vi "CtrlTrain_Analog_Scale.vi"(4 "Raw_High":dbl=5.0, 6 "Raw_Low":dbl, 8 "Out_Low":dbl, 9 "Out_High":dbl=100.0, 11 "Input":dbl) -> (0 "B":dbl, 1 "M":dbl, 3 "Output":dbl)   [LabVIEW 2019, in "CtrlTrainingLibary_Protected.lvlib"]
doc: "This VI rate limits the input. This VI remembers the last output. If there are multiple VI that set the same output, use the RateLimit2 VI. This one has an input connection to send the last output value."
uses:
  CtrlTrainingLibary_Protected.lvlib
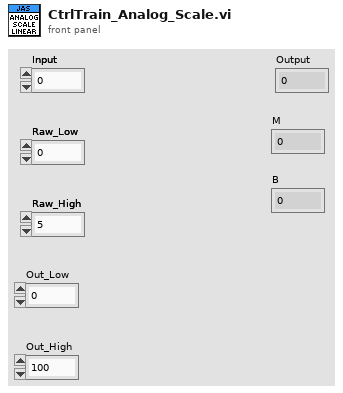
[diagram p1: front panel]
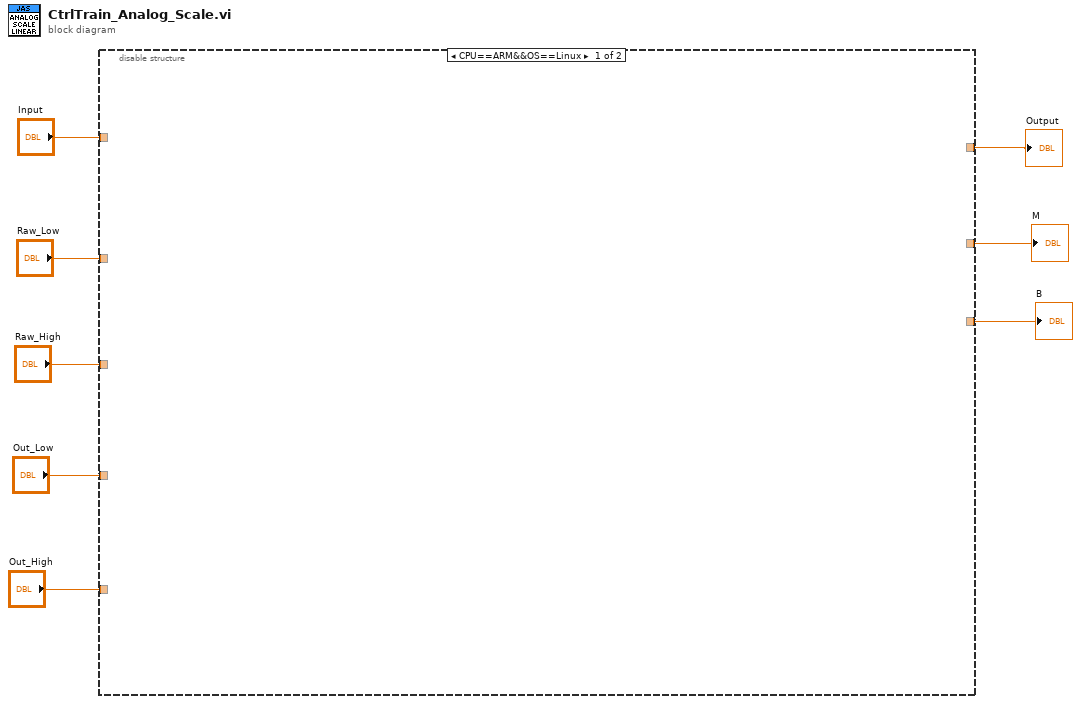
[diagram p0: block diagram]
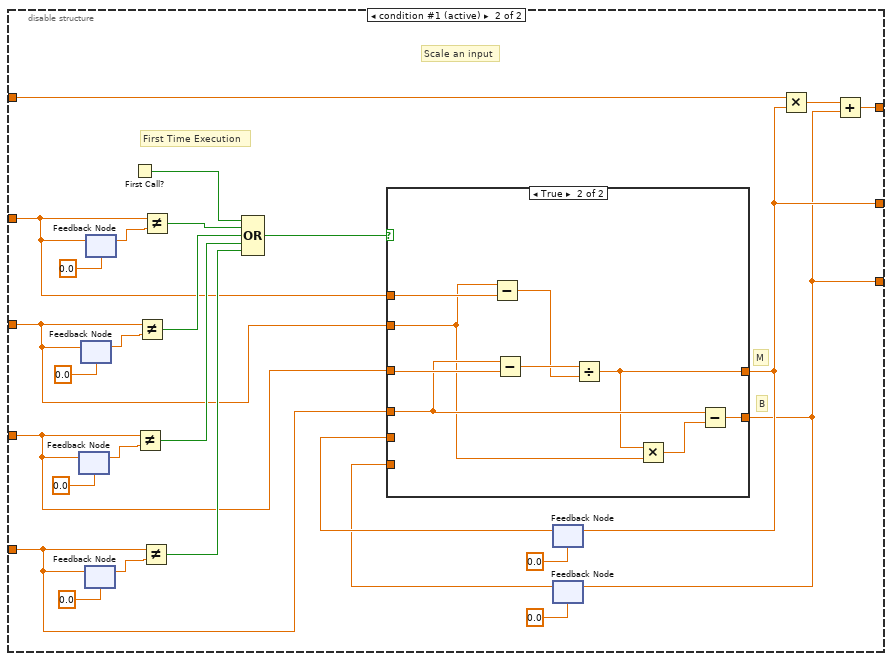
[diagram p2: hidden frame]
diagram:
  n1 = disable-structure shown="CPU==ARM&&OS==Linux" {
    disable-tunnel: "Raw_Low" -> [_ w22]
    disable-tunnel: "Raw_High" -> [_ w21]
    disable-tunnel: "Out_Low" -> [_ w20]
    disable-tunnel: "Out_High" -> [_ w19]
    disable-tunnel: "Input" -> [_ w18]
    disable-tunnel: [_ w16] -> w3
    disable-tunnel: [_ w13] -> w2
    disable-tunnel: [_ w10] -> w1
    frame condition #0 {
    }
    frame condition #1 (active) {
      # "First Time Execution"
      # "Scale an input"
      # "B"
      # "M"
      n2 = feedback #1(0.0 ("Raw_Low")) -> (w31:dbl)
      n3 = feedback-in #1(w20) -> ()
      n4 = feedback #2(0.0 ("Raw_Low")) -> (w33:dbl)
      n5 = feedback-in #2(w21) -> ()
      n6 = feedback #3(0.0 ("Raw_Low")) -> (w29:dbl)
      n7 = feedback-in #3(w19) -> ()
      n8 = feedback #4(0.0 ("Raw_Low")) -> (w35:dbl)
      n9 = feedback-in #4(w22) -> ()
      n10 = First Call?() -> (First Call?: T/F=w9:bool)
      n11 = Not Equal?(x=w20, y=w31) -> (x != y?=w25:bool)
      n12 = Not Equal?(x=w21, y=w33) -> (x != y?=w26:bool)
      n13 = Not Equal?(x=w19, y=w29) -> (x != y?=w24:bool)
      n14 = Not Equal?(x=w22, y=w35) -> (x != y?=w27:bool)
      n15 = Compound Arithmetic op=OR(w9, w27, w26, w25, w24) -> (w23:bool)
      n16 = feedback #5(0.0) -> (w12:dbl)
      n17 = feedback #6(0.0) -> (w11:dbl)
      n18 = case shown="True" w23 {
        tunnel: w22 -> [_ w45]
        tunnel: w21 -> [_ w41]
        tunnel: w20 -> [_ w46]
        tunnel: w19 -> [_ w42]
        tunnel: [w37 w39] -> w16
        tunnel: [w36 w38] -> w13
        tunnel: w12 -> [w37 _]
        tunnel: w11 -> [w36 _]
        frame False {
        }
        frame True {
          n19 = Subtract(x=w41, y=w45) -> (x-y=w43:dbl)
          n20 = Subtract(x=w42, y=w46) -> (x-y=w44:dbl)
          n21 = Divide(x=w44, y=w43) -> (x/y=w39:dbl)
          n22 = Multiply(x=w39, y=w41) -> (x*y=w40:dbl)
          n23 = Subtract(x=w42, y=w40) -> (x-y=w38:dbl)
        }
      }
      n24 = feedback-in #5(w16) -> ()
      n25 = feedback-in #6(w13) -> ()
      n26 = Multiply(x=w18, y=w16) -> (x*y=w17:dbl)
      n27 = Add(x=w17, y=w13) -> (x+y=w10:dbl)
    }
  }
  "Output" <- w1
  "M" <- w3
  "B" <- w2
